vi "main.vi"   [LabVIEW 2017]
uses:
  globalUtilities.vi
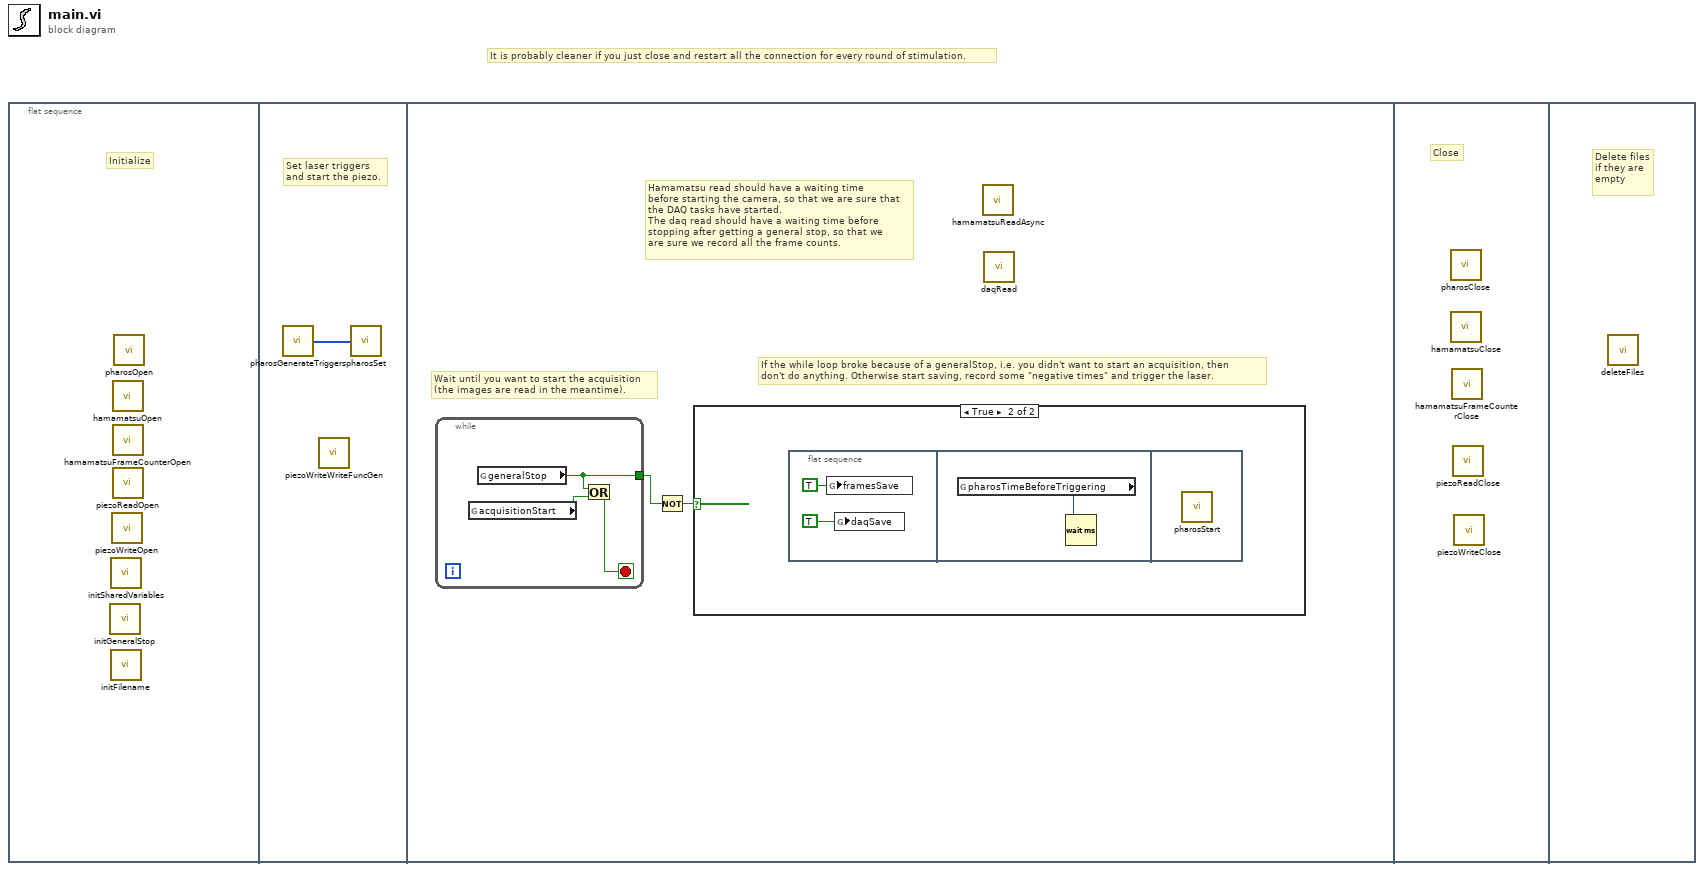
[diagram p0: block diagram]
diagram:
  # "It is probably cleaner if you just close and restart all the connection for every round of stimulation."
  n1 = flat-sequence {
    frame #0 {
      # "Initialize"
      n2 = call "initGeneralStop.vi"() -> ()  [unwired: 1 in]
      n3 = call "initSharedVariables.vi"() -> ()  [unwired: 12 in]
      n4 = call "initFilename.vi"() -> ()  [unwired: 2 in, 1 out]
      n5 = call "piezoWriteOpen.vi"() -> ()  [unwired: 2 in]
      n6 = call "hamamatsuOpen.vi"() -> ()  [unwired: 4 out]
      n7 = call "hamamatsuFrameCounterOpen.vi"() -> ()  [unwired: 12 in]
      n8 = call "piezoReadOpen.vi"() -> ()  [unwired: 6 in]
      n9 = call "pharosOpen.vi"() -> ()  [unwired: 1 in]
    }
    frame #1 {
      # "Set laser triggers\nand start the piezo."
      n10 = call "pharosGenerateTriggers.vi"() -> ("triggers"=w1:u8[])  [unwired: 1 in]
      n11 = call "piezoWriteWriteFuncGen.vi"() -> ()  [unwired: 12 in]
      n12 = call "pharosSet.vi"("triggers"=w1) -> ()
    }
    frame #2 {
      # "Hamamatsu read should have a waiting time\nbefore starting the camera, so that we are sure that\nthe DAQ tasks have started.\nThe daq read should have a waiting time before\nstopping after getting a general stop, so that we\nare sure we record all the frame counts."
      # "If the while loop broke because of a generalStop, i.e. you didn't want to start an acquisition, then\ndon't do anything. Otherwise start saving, record some \"negative times\" and trigger the laser."
      # "Wait until you want to start the acquisition\n(the images are read in the meantime)."
      n13 = while {
        tunnel: [w7] -> w2
        stop <- w8 stop-if-true
        n14 = global read "globalUtilities.vi" "acquisitionStart"() -> (w9:bool)
        n15 = global read "globalUtilities.vi" "generalStop"() -> (w7:bool)
        n16 = Or(x=w7, y=w9) -> (x .or. y?=w8:bool)
      }
      n17 = Not(x=w2) -> (.not. x?=w3:bool)
      n18 = case shown="True" w3 {
        frame False {
        }
        frame True {
          n19 = flat-sequence {
            frame #0 {
              n20 = global write "globalUtilities.vi" "framesSave"(TRUE ("framesSave")) -> ()
              n21 = global write "globalUtilities.vi" "daqSave"(TRUE ("framesSave")) -> ()
            }
            frame #1 {
              n22 = global read "globalUtilities.vi" "pharosTimeBeforeTriggering"() -> (w6:u32)
              n23 = Wait (ms)(milliseconds to wait=w6) -> ()  [unwired: 1 out]
            }
            frame #2 {
              n24 = call "pharosStart.vi"() -> ()  [unwired: 12 in]
            }
          }
        }
      }
      n25 = call "hamamatsuReadAsync.vi"() -> ()  [unwired: 12 in]
      n26 = call "daqRead.vi"() -> ()  [unwired: 3 in]
    }
    frame #3 {
      # "Close"
      n27 = call "pharosClose.vi"() -> ()  [unwired: 12 in]
      n28 = call "hamamatsuClose.vi"() -> ()  [unwired: 1 out]
      n29 = call "hamamatsuFrameCounterClose.vi"() -> ()  [unwired: 12 in]
      n30 = call "piezoReadClose.vi"() -> ()  [unwired: 1 in]
      n31 = call "piezoWriteClose.vi"() -> ()  [unwired: 1 in]
    }
    frame #4 {
      # "Delete files\nif they are\nempty"
      n32 = call "deleteFiles.vi"() -> ()  [unwired: 12 in]
    }
  }
